vi "Actor Core.vi"(8 "error in (no error)":errorcluster, 11 "WSClient-P40001 in":refnum<class "WS Client.lvclass">) -> (0 "error out":errorcluster, 3 "Mediated Asynchronous Actor out":refnum<class "WS Client.lvclass">)   [LabVIEW 2016, in "WebSocket Networking.lvlib" / "WS Client.lvclass"]
doc: "--\nCopyright © 2017 Composed SystemsI All rights reserved.\n\nAuthor: Jon McBee <jon.mcbee@composed.io>\n\nThis library is provided \"AS IS\" ,WITHOUT WARRANTIES OR\nCONDITIONS OF ANY KIND, either express or implied.\n\nComposed Systems -- composed.io\n\nStream 0.0.1.1\nJon McBee - Composed Systems\nCopyright (c) 2017, Composed Systems"
uses:
  <userlib>/Common Components/WebSocket Networking/WS Client/WS Client.lvclass
  C:/Program Files (x86)/National Instruments/LabVIEW 2016/user.lib/Composed Systems/Stream/Mediator/Classes/Mediated Asynchronous Actor/Mediated Asynchronous Actor.lvclass
  C:/Program Files (x86)/National Instruments/LabVIEW 2016/user.lib/Composed Systems/Stream/Mediator/Classes/Websocket Client Handler Actor/Websocket Client Handler/Websocket Client Handler.lvclass
  <userlib>/Common Components/WebSocket Networking/WS Client/WS Client.lvclass/WS Client.ctl
  <userlib>/Composed Systems/Stream/Mediator/Classes/Websocket Client Handler Actor/Websocket Client Handler/Websocket Client Handler.lvclass
  <userlib>/Composed Systems/Stream/Mediator/Classes/Mediated Asynchronous Actor/Mediated Asynchronous Actor.lvclass
  <userlib>/Common Components/WebSocket Networking/WS Server Msgs/Add Connected Client to WSserver Msg/Add Connected Client to WSserver Msg.lvclass
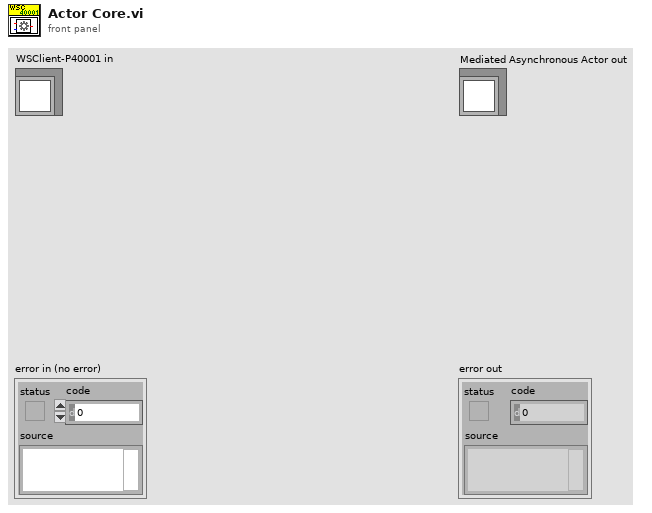
[diagram p1: front panel]
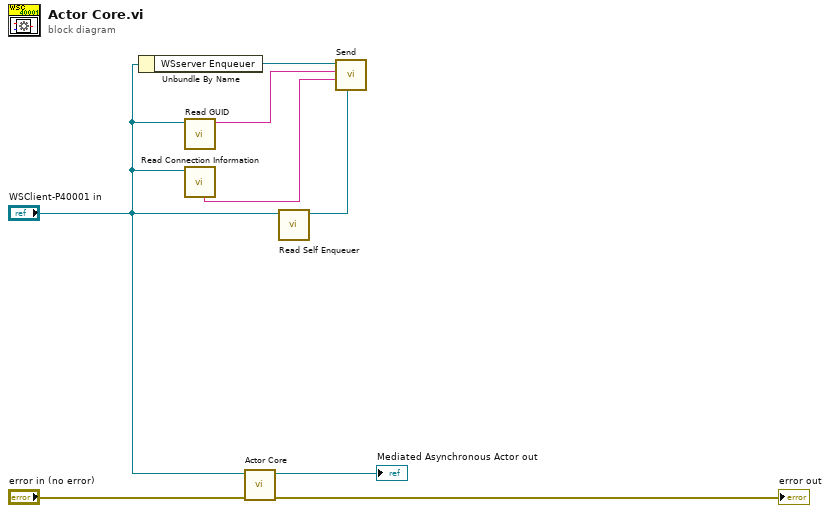
[diagram p0: block diagram]
diagram:
  n1 = Unbundle By Name("WSClient-P40001 in") -> ("WSserver Enqueuer"=w5:refnum<class "Message Transport Queue.lvclass">)
  n2 = call <userlib>:"Read GUID.vi"("Mediated Asynchronous Actor in"="WSClient-P40001 in") -> ("GUID"=w4:string)  [unwired: 10 in]
  n3 = call <userlib>:"Read Connection Information.vi"("Websocket Client Handler in"="WSClient-P40001 in") -> ("Remote Address"=w2:string)  [unwired: 8 in, 2 out]
  n4 = call-parent "Actor Core.vi"("error in (no error)"="error in (no error)", "Websocket Client Handler in"="WSClient-P40001 in") -> ("error out"=→"error out":errorcluster, "Mediated Asynchronous Actor out"=→"Mediated Asynchronous Actor out":refnum<class "WS Client.lvclass">)  [unwired: 8 in]
  n5 = call <userlib>:"Read Self Enqueuer.vi"("Mediated Asynchronous Actor in"="WSClient-P40001 in") -> ("Self Enqueuer"=w1:refnum<class "Message Transport Queue.lvclass">)  [unwired: 10 in]
  n6 = call <userlib>:"Send.vi"("Websocket Client Handler MTQ"=w1, "IP Address"=w2, "GUID"=w4, "Message Transport Queue"=w5) -> ()  [unwired: 7 in, 1 out]
